vi "StartTopicServer.vi"(2 "Baxter in":T1, 3 "Registration":enum16{"Register", "Unregister"}(ring)) -> (0 "Baxter out":T1)   [LabVIEW 2013]
uses:
  _ROSControl.ctl
  _ROSDirection.ctl
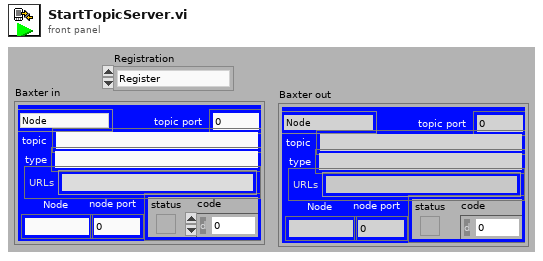
[diagram p1: front panel]
types:
  T1 = typedef "_ROSControl.ctl" = cluster{"topic port":u16, "Node":string, "topic":string, "type":string, "node port":u32, "error ":errorcluster, "Direction":T2, "APIs":string[]}
  T2 = typedef "_ROSDirection.ctl" = enum16{"Node", "Publisher", "Subscriber", "Service Client"}
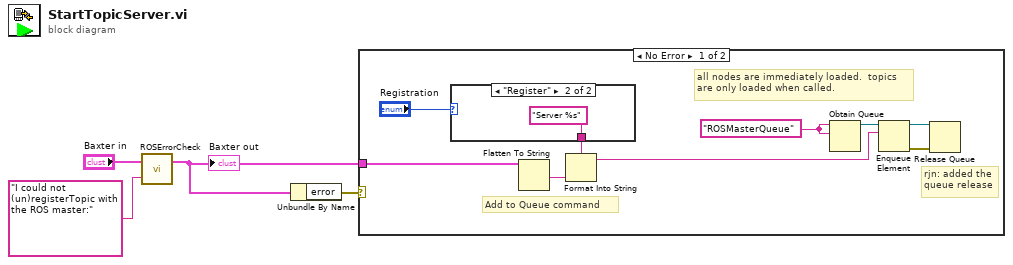
[diagram p0: block diagram]
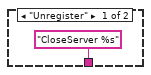
[diagram p2: hidden frame]
diagram:
  n1 = call "ROSErrorCheck.vi"("message"="I could not (un)registerTopic with the ROS master:", "ROS in"="Baxter in") -> ("ROS out"=w1:T1)  [unwired: 1 in]
  "Baxter out" <- w1
  n2 = Unbundle By Name(w1) -> ("error"=w4:errorcluster)
  n3 = case shown="No Error" w4 {
    tunnel: w1 -> [w8 _]
    frame No Error {
      w9 = "ROSMasterQueue" ("name (unnamed)")
      # "rjn: added the\nqueue release"
      # "Add to Queue command"
      # "all nodes are immediately loaded.  topics\nare only loaded when called."
      n4 = case shown="\"Register\"" "Registration" {
        tunnel: ["CloseServer %s" ("format string") "Server %s" ("format string")] -> w12
        frame "Unregister" {
        }
        frame "Register" {
        }
      }
      n5 = Flatten To String(anything=w8) -> (data string=w7:string)  [unwired: 3 in, 2 out]
      n6 = Format Into String(format string=w12, w7) -> (resulting string=w11:string)  [unwired: 2 in, 1 out]
      n7 = Obtain Queue(name (unnamed)=w9, element data type=w9) -> (queue out=w10:refnum<queue>)  [unwired: 3 in, 2 out]
      n8 = Enqueue Element(queue=w10, element=w11) -> (queue out=w6:refnum<queue>, error out=w5:errorcluster)  [unwired: 2 in, 1 out]
      n9 = Release Queue(queue=w6, error in (no error)=w5) -> ()  [unwired: 1 in, 3 out]
    }
    frame Error {
    }
  }
